vi "AIM664 Board Control.vi"() -> ()   [LabVIEW 2020]
uses:
  examples/bsp/typedefs/BoardControlIn.ctl
  AIM664LV.lvlib
panel:
  in  "ResourceID":u32=1
  out "ARINC 664 Resources":string[](tree)
  out "Output Parameters":T1 {"SharedMemFree" format="%x"; "GlobalMemFree" format="%x"; "ExpertMode" items=["FDX_EXPERT_MODE", "FDX_DISA_GHOST"]; "PortGoodLink" items=["FDX_NO_LINK", "FDX_GOOD_LINK"]; "PortSpeed" items=["FDX_100MBIT", "FDX_10MBIT", "FDX_AUTO_100MBIT", "FDX_AUTO_10MBIT"]; "PortConfig" items=["FDX_SINGLE", "FDX_REDUNDANT"]}
  in  "Input Parameters":T2 {"Expert4Mode" items=["FDX_EXPERT_MODE", "FDX_DISA_GHOST"]; "Expert3Mode" items=["FDX_EXPERT_MODE", "FDX_DISA_GHOST"]; "Expert2Mode" items=["FDX_EXPERT_MODE", "FDX_DISA_GHOST"]; "Expert1Mode" items=["FDX_EXPERT_MODE", "FDX_DISA_GHOST"]; "Port4SpeedIn" items=["FDX_100MBIT", "FDX_10MBIT", "FDX_AUTO_100MBIT", "FDX_AUTO_10MBIT"]; "Port3SpeedIn" items=["FDX_100MBIT", "FDX_10MBIT", "FDX_AUTO_100MBIT", "FDX_AUTO_10MBIT"]; "Port2SpeedIn" items=["FDX_100MBIT", "FDX_10MBIT", "FDX_AUTO_100MBIT", "FDX_AUTO_10MBIT"]; "Port1SpeedIn" items=["FDX_100MBIT", "FDX_10MBIT", "FDX_AUTO_100MBIT", "FDX_AUTO_10MBIT"]; "Port4ConfigIn" items=["FDX_SINGLE", "FDX_REDUNDANT"]; "Port3ConfigIn" items=["FDX_SINGLE", "FDX_REDUNDANT"]; "Port2ConfigIn" items=["FDX_SINGLE", "FDX_REDUNDANT"]; "Port1ConfigIn" items=["FDX_SINGLE", "FDX_REDUNDANT"]; "Control" items=["FDX_READ", "FDX_WRITE"]}
  out "NuOfResources":u32
  in  "Server Name":string="local"
  out "Number of Servers":u32=1
  # "ARINC 664 Board Control"
  # "Overview: Queries the boards available in a system and present some properties of those resources.\nRequirement: At least one AIM ARINC-664 board with installed AIM ARINC 664 BSP.\nRestrictions: None.\nInstruction:\n1. Run the VI.\n2. Verify the resources available. If no error is presented, you will see all of the resources in the Resources."
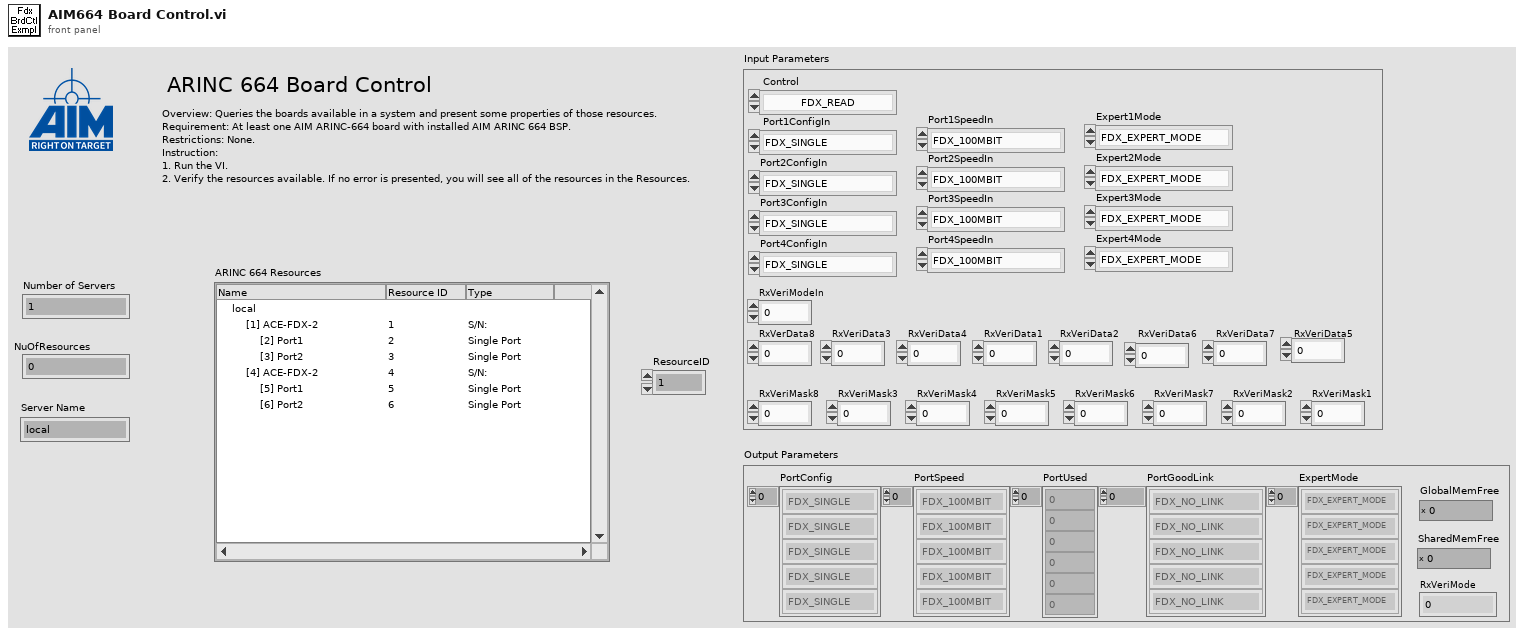
[diagram p1: front panel]
types:
  T1 = cluster{"PortConfig":u32[], "PortSpeed":u32[], "PortUsed":u32[], "PortGoodLink":u32[], "ExpertMode":u32[], "GlobalMemFree":u32, "SharedMemFree":u32, "RxVeriMode":u32}
  T2 = typedef "BoardControlIn.ctl" = cluster{"Control":u32, "Port1ConfigIn":u32, "Port2ConfigIn":u32, "Port3ConfigIn":u32, "Port4ConfigIn":i32, "Port1SpeedIn":u32, "Port2SpeedIn":u32, "Port3SpeedIn":u32, "Port4SpeedIn":u32, "Expert1Mode":u32, "Expert2Mode":u32, "Expert3Mode":u32, "Expert4Mode":u32, "RxVeriModeIn":u32, "RxVeriData1":u32, "RxVeriData2":u32, "RxVeriData3":u32, "RxVeriData4":u32, "RxVeriData5":u32, "RxVeriData6":u32, "RxVeriData7":u32, "RxVeriMask1":u32, "RxVeriMask2":u32, "RxVeriMask3":u32, "RxVeriMask4":u32, "RxVeriMask5":u32, "RxVeriMask6":u32, "RxVeriMask7":u32, "RxVerData8":u32, "RxVeriMask8":u32}
  T3 = cluster{"BoardName":string, "BoardSerialNo":u32, "BoardNumOf\nEthernetPorts":u32, "BoardClients":u32, "BoardGlobal\nMemSize":u32, "BoardShared\nMemSize":u32, "BoardStructId":u32, "PortName":string, "PortMode":u32, "PortNo":u32, "PortBoard\nResourceID":u32, "PortStructId":u32}
  T4 = cluster{"Left Cell String":string, "Child Text":string[], "Child Tag":string, "Item Indent":i32, "Child Only?":bool, "Glyph Index":i32}
  T5 = cluster{"Left Cell String":string, "Child Text":string[], "Child Tag":string, "Item Indent":i32, "Child Only?":bool, "Glyph Index":i32}[]
  T6 = typedef "AIM664LV.lvlib/port_configuration.ctl" = u32
  T7 = typedef "AIM664LV.lvlib/port_speed.ctl" = u32
  T8 = typedef "AIM664LV.lvlib/port_condition.ctl" = u32
  T9 = typedef "AIM664LV.lvlib/expert_mode.ctl" = u32
  T10 = cluster{"PortConfig":T6[], "PortSpeed":T7[], "PortUsed":u32[], "PortGoodLink":T8[], "ExpertMode":T9[], "GlobalMemFree":u32, "SharedMemFree":u32, "RxVeriMode":u32}
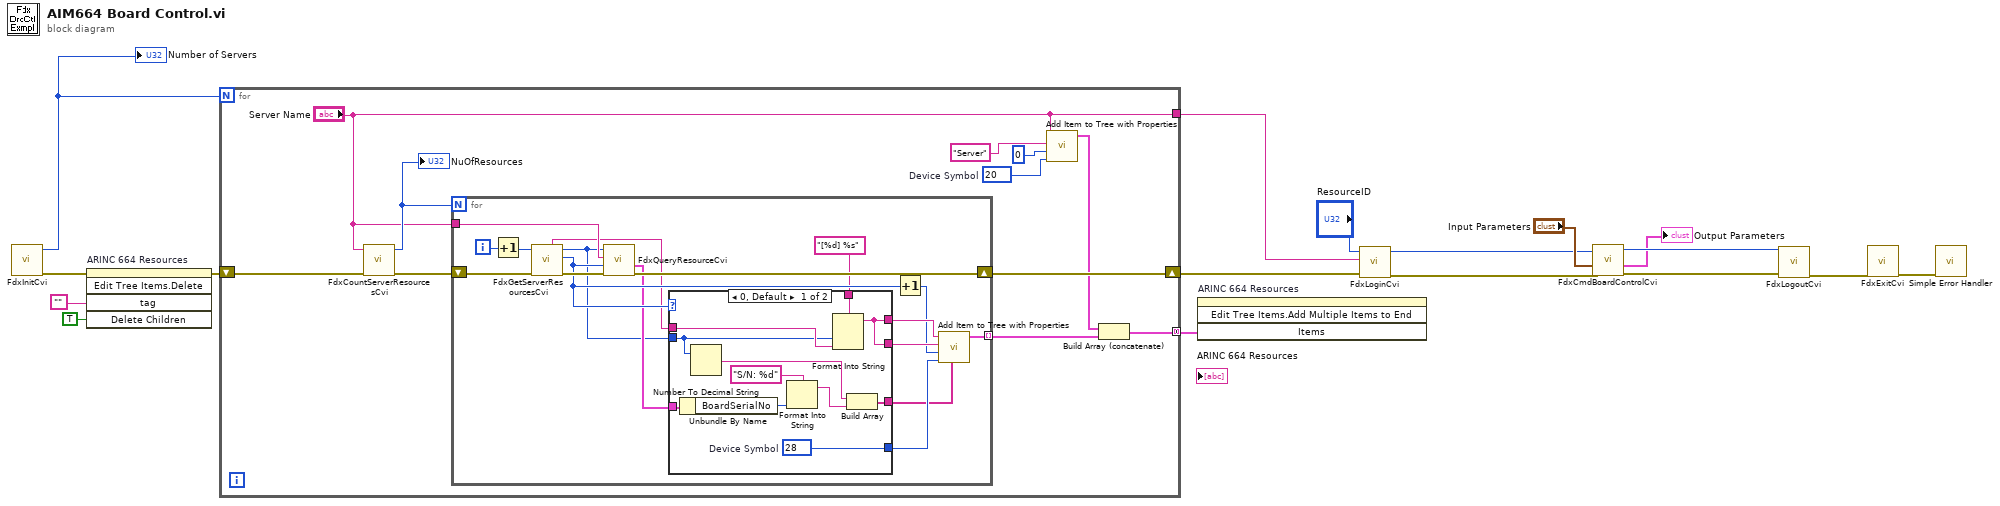
[diagram p0: block diagram]
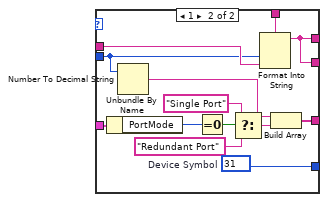
[diagram p2: hidden frame]
diagram:
  n1 = call "FdxInitCvi.vi"() -> ("error out"=w7:errorcluster, "Number of Servers"=w9:u32)  [unwired: 10 in]
  "Number of Servers" <- w9
  n2 = invoke on="ARINC 664 Resources" class="Tree (strict)" method="Edit Tree Items.Delete"(error in=w7, "tag"="", "Delete Children"=TRUE ("Delete Children?")) -> (error out=w6:errorcluster)  [unwired: 2 in, 4 out]
  n3 = for {
    N: w9 -> [_]
    shift-right: [w26] -> w17
    shift-left: w6 -> [w28]
    tunnel: [w23] -> w8 mode=concatenating
    tunnel: ["Server Name"] -> w3
    w21 = 20  # Device Symbol
    n4 = call "FdxCountServerResourcesCvi.vi"("error in"=w28, "SrvName (local)"="Server Name") -> ("error out"=w27:errorcluster, "Number of Resources"=w25:u32)  [unwired: 8 in]
    "NuOfResources" <- w25
    n5 = for {
      N: w25 -> [_]
      shift-right: [w38] -> w26
      shift-left: w27 -> [w45]
      tunnel: [w42] -> w24 mode=indexing
      tunnel: "Server Name" -> [w37]
      i -> [w43]
      n6 = Increment(x=w43) -> (x+1=w40:i32)
      n7 = call "FdxGetServerResourcesCvi.vi"("error in"=w45, "ServerRElement"=w40) -> ("error out"=w39:errorcluster, "ResourceType"=w36:u32, "Resource ID"=w33:u32, "Resource Info"=w34:string)  [unwired: 4 in, 2 out]
      n8 = call "FdxQueryResourceCvi.vi"("error in"=w39, "ResourceType"=w36, "SrvName"=w37, "ResourceID"=w33) -> ("error out"=w38:errorcluster, "ResourceInfo"=w35:T3)  [unwired: 5 in, 1 out]
      n9 = case shown="0, Default" w36 {
        tunnel: [w56 w69] -> w44
        tunnel: [w48 w59] -> w41
        tunnel: w35 -> [w53 w66]
        tunnel: w34 -> [w55 w67]
        tunnel: w33 -> [w47 w57]
        tunnel: [w48 w59] -> w32
        tunnel: "[%d] %s" ("format string") -> [w54 w68]
        tunnel: [w52 w60] -> w30
        frame 0, Default {
          w56 = 28  # Device Symbol
          n10 = Unbundle By Name(w53) -> ("BoardSerialNo"=w51:u32)
          n11 = Number To Decimal String(number=w47) -> (decimal integer string=w46:string)  [unwired: 1 in]
          n12 = Format Into String(format string="S/N: %d", w51) -> (resulting string=w50:string)  [unwired: 2 in, 1 out]
          n13 = Format Into String(format string=w54, w47, w55) -> (resulting string=w48:string)  [unwired: 2 in, 1 out]
          n14 = Build Array(w46, w50) -> (w52:string[])
        }
        frame 1 {
          w69 = 31  # Device Symbol
          n15 = Unbundle By Name(w66) -> ("PortMode"=w65:u32)
          n16 = Number To Decimal String(number=w57) -> (decimal integer string=w58:string)  [unwired: 1 in]
          n17 = Equal To 0?(x=w65) -> (x = 0?=w64:bool)
          n18 = Select(t="Single Port" ("Child Tag"), s=w64, f="Redundant Port" ("Child Tag")) -> (s? t:f=w63:string)
          n19 = Format Into String(format string=w68, w57, w67) -> (resulting string=w59:string)  [unwired: 2 in, 1 out]
          n20 = Build Array(w58, w63) -> (w60:string[])
        }
      }
      n21 = Increment(x=w36) -> (x+1=w29:u32)
      n22 = call "Add Item to Tree with Properties.vi"("Child Text"=w30, "Glyph Index"=w44, "Item indent"=w29, "Child Tag"=w41, "Left Cell String"=w32) -> ("Item"=w42:T4)  [unwired: 6 in]
    }
    n23 = call "Add Item to Tree with Properties.vi"("Glyph Index"=w21, "Item indent"=0, "Child Tag"="Server", "Left Cell String"="Server Name") -> ("Item"=w22:T4)  [unwired: 7 in]
    n24 = Build Array (concatenate)(w22, w24) -> (w23:T5)
  }
  n25 = invoke on="ARINC 664 Resources" class="Tree (strict)" method="Edit Tree Items.Add Multiple Items to End"("Items"=w8) -> ()  [unwired: 3 in, 4 out]
  n26 = call "FdxLoginCvi.vi"("error in"=w17, "SrvName"=w3, "ResourceID"="ResourceID") -> ("error out"=w11:errorcluster, "InstrumentHandle"=w10:u32)  [unwired: 7 in]
  n27 = call "FdxCmdBoardControlCvi.vi"("error in"=w11, "BoardControlIn (read)"="Input Parameters", "InstrumentHandle_board in"=w10) -> ("error out"=w16:errorcluster, "Board Control Out"=→"Output Parameters":T10, "InstrumentHandle_board out"=w14:u32)  [unwired: 6 in]
  n28 = call "FdxLogoutCvi.vi"("error in"=w16, "InstrumentHandle"=w14) -> ("error out"=w15:errorcluster)  [unwired: 9 in]
  n29 = call "FdxExitCvi.vi"("error in"=w15) -> ("error out"=w1:errorcluster)  [unwired: 10 in]
  n30 = call <vilib>:"Simple Error Handler.vi"("error in (no error)"=w1) -> ()  [unwired: 4 in, 5 out]
